vi "Get FPS.vi"(0 "comm interface in":refnum<class "Pixy Com.lvclass">, 11 "error in":errorcluster) -> (4 "comm interface out":refnum<class "Pixy Com.lvclass">, 6 "fps":u32, 15 "error out":errorcluster)   [LabVIEW 2018, in "Pixy2.lvlib"]
doc: "Gets Pixy2's current frames-per-second."
uses:
  Interface/Pixy Com.lvclass
  Pixy2.lvlib
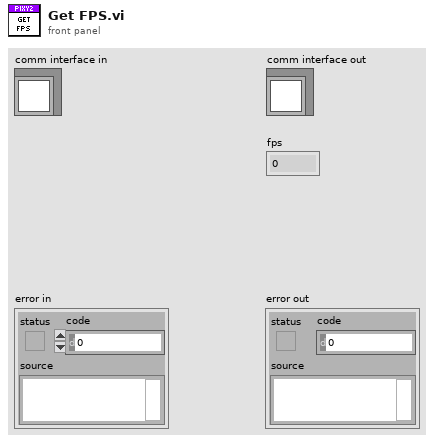
[diagram p1: front panel]
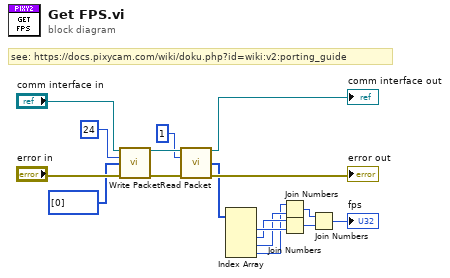
[diagram p0: block diagram]
diagram:
  # "see: https://docs.pixycam.com/wiki/doku.php?id=wiki:v2:porting_guide"
  n1 = call "Write Packet.vi"("comm interface in"="comm interface in", "type"=u8 24, "payload"=u8[] [0], "error in"="error in") -> ("comm interface out"=w14:refnum<class "Pixy Com.lvclass">, "error out"=w15:errorcluster)  [unwired: 10 in]
  n2 = call "Read Packet.vi"("comm interface in"=w14, "expected type"=u8 1, "error in"=w15) -> ("comm interface out"=→"comm interface out":refnum<class "Pixy Com.lvclass">, "received"=w8:u8[], "error out"=→"error out":errorcluster)  [unwired: 9 in, 1 out]
  n3 = Index Array(array=w8) -> (element #1=w7:u8, element #2=w4:u8, element #3=w3:u8, element #4=w2:u8)  [unwired: 4 in]
  n4 = Join Numbers(hi=w2, lo=w3) -> ((hi.lo)=w5:u16)
  n5 = Join Numbers(hi=w4, lo=w7) -> ((hi.lo)=w6:u16)
  n6 = Join Numbers(hi=w5, lo=w6) -> ((hi.lo)=→"fps":u32)
